vi "Set Shutter Status.vi"(8 "error in (no error)":errorcluster {"code" format="%.0x"}, 9 "Shutter Status (0: Open)":enum16{"Open", "Close"}(ring), 10 "Device Number (1)":i32=1, 11 "VISA Resource Name":refnum<visa-resource-name>) -> (0 "error out":errorcluster {"code" format="%.0x"}, 3 "VISA Resource Name Out":refnum<visa-resource-name>)   [LabVIEW 2020, in "Olympus IX BX Series.lvlib"]
doc: "Controls the shutter (RFAA).\n\nNotes:\n(1) This VI is valid only for Olympus BX2A model."
uses:
  Olympus IX BX Series.lvlib
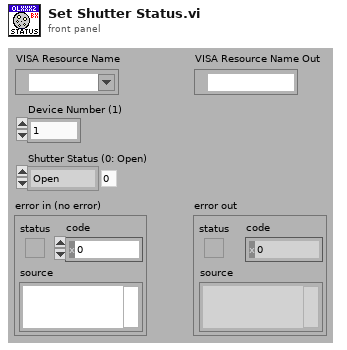
[diagram p1: front panel]
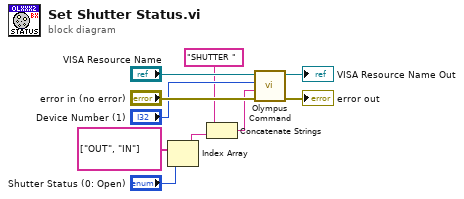
[diagram p0: block diagram]
diagram:
  n1 = Index Array(array=string[] ["OUT", "IN"], index="Shutter Status (0: Open)") -> (element=w3:string)
  n2 = Concatenate Strings("SHUTTER " ("format string"), w3) -> (w1:string)
  n3 = call "Olympus Command.vi"("error in (no error)"="error in (no error)", "Command string"=w1, "Device Number (1)"="Device Number (1)", "VISA Resource Name"="VISA Resource Name") -> ("error out"=→"error out":errorcluster, "VISA Resource Name Out"=→"VISA Resource Name Out":refnum<visa-resource-name>)  [unwired: 5 in, 1 out]
